vi "Rectangle_Create.vi"(8 "Error In":errorcluster, 9 "H":i32, 10 "W":i32, 11 "reference in":refnum<class "Rectangle.lvclass">) -> (0 "Error Out":errorcluster, 3 "reference out":refnum<class "Rectangle.lvclass">)   [LabVIEW 2020, in "Rectangle.lvclass"]
uses:
  Rectangle.lvclass
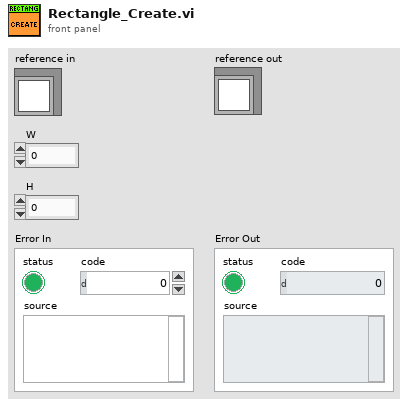
[diagram p1: front panel]
types:
  T1 = typedef "Rectangle.lvclass/ObjectAttributes.ctl" = cluster{"_width":i32, "_height":i32}
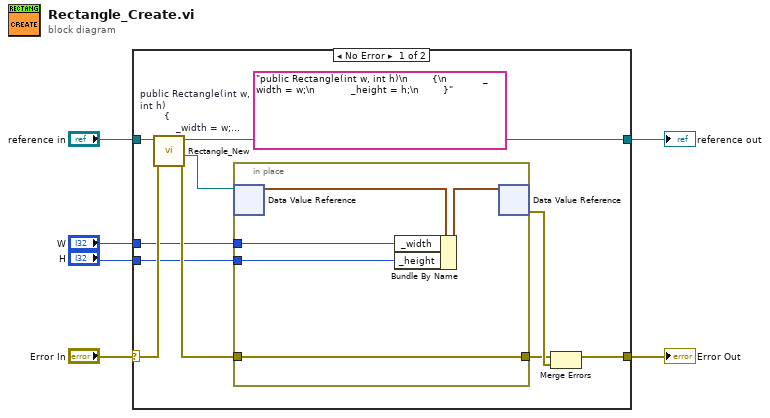
[diagram p0: block diagram]
diagram:
  n1 = case shown="No Error" "Error In" {
    selector: "Error In" -> [w15 w23]
    tunnel: [w9 w23] -> w5
    tunnel: "reference in" -> [w16 w22]
    tunnel: [w14 w22] -> w3
    tunnel: "W" -> [w8 _]
    tunnel: "H" -> [w7 _]
    frame No Error {
      (unwired) "public Rectangle(int w, int h)\n        {\n            _width = w;\n            _height = h;\n        }"  # public Rectangle(int w, int h)         {             _width = w;             _height = h;         }
      n2 = call "Rectangle_New.vi"("error in (no error)"=w15, "reference in"=w16) -> ("error out"=w11:errorcluster, "DVRRefOut"=w12:refnum<data-value>, "reference out"=w14:refnum<class "Rectangle.lvclass">)  [unwired: 6 in, 1 out]
      n3 = in-place {
        in-place-border: w11 -> [w19]
        in-place-border: [w19] -> w10
        in-place-border: w8 -> [w18]
        in-place-border: w7 -> [w17]
        n4 = in-place-dvr #1(w12) -> (w20:T1)  [unwired: 1 out]
        n5 = Bundle By Name(cluster=w20, "_width"=w18, "_height"=w17) -> (w21:T1)
        n6 = in-place-dvr #1(w21) -> (w13:errorcluster)  [unwired: 1 out]
      }
      n7 = Merge Errors(w10, w13) -> (w9:errorcluster)
    }
    frame Error {
      # "VI-TechBaseTemplate_Simple_4x4x4"
    }
  }
  "Error Out" <- w5
  "reference out" <- w3
